vi "DataCSVFileRichInfo.vi"(9 "Language":u32, 11 "file path (dialog if empty)":path caption="文件路径 （空时为对话框）") -> (0 "路径输出":path, 1 "FileInfo":string, 2 "文件类型":string)   [LabVIEW 2015]
uses:
  <vilib>/regexp/Match Regular Expression.xnode
panel:
  out "判断":string
  out "末行":string
  out "数据首行":string
  out "行首":string
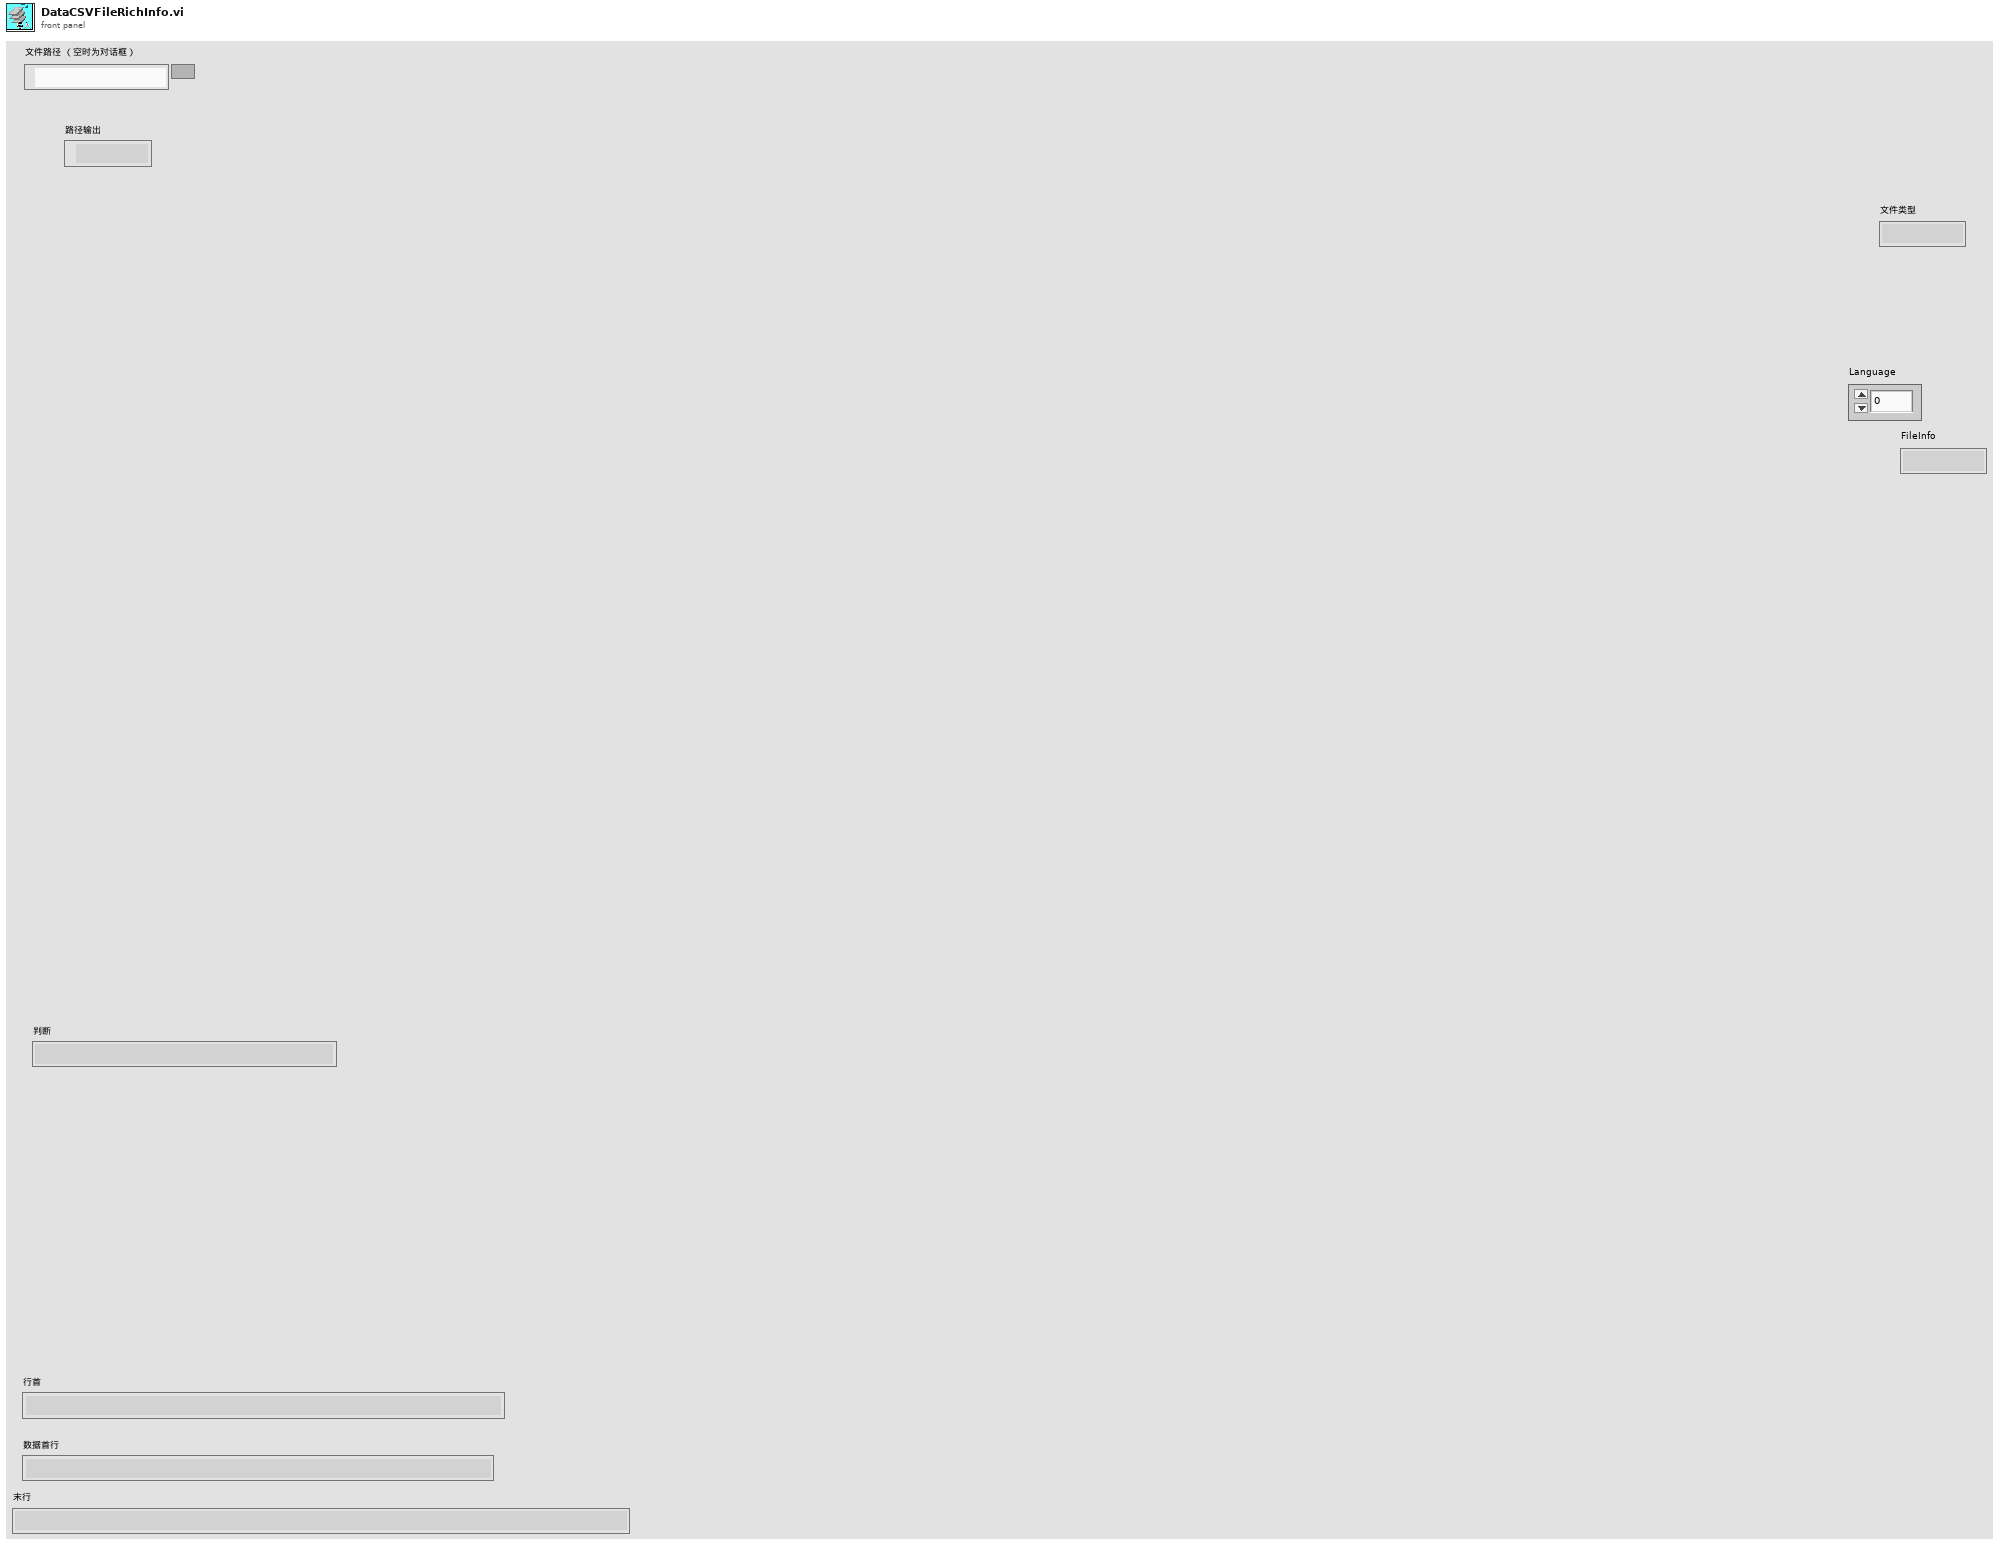
[diagram p1: front panel]
types:
  T1 = cluster{"基时间字符串":string, "基时间秒":dbl, "基时间标识":timestamp}
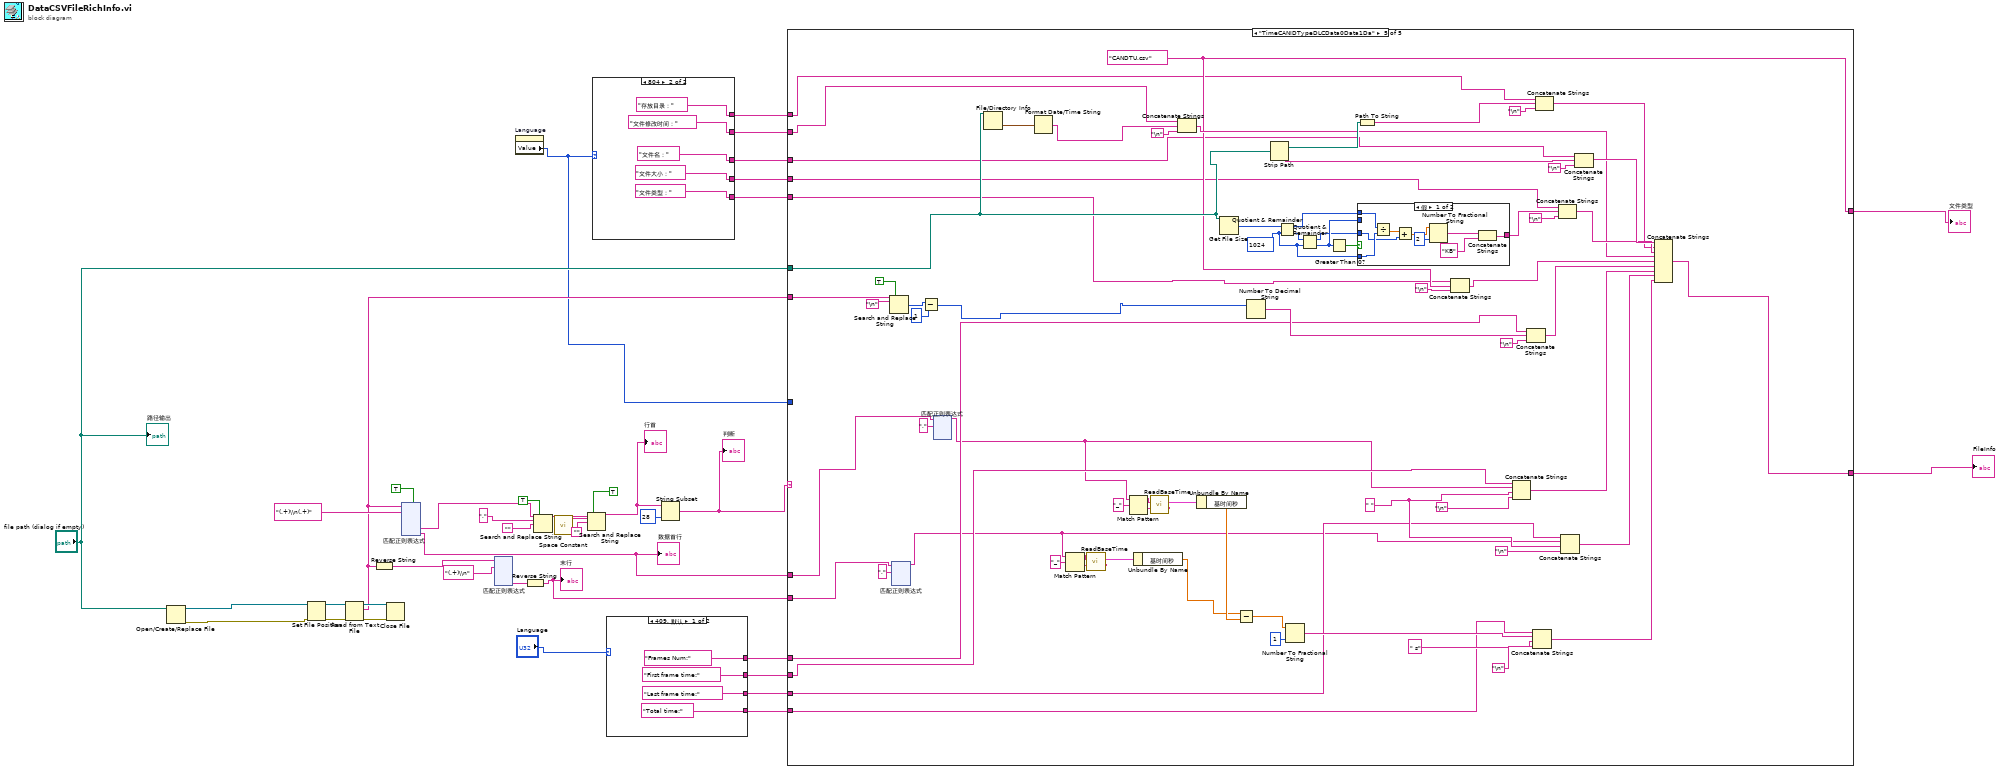
[diagram p0: block diagram]
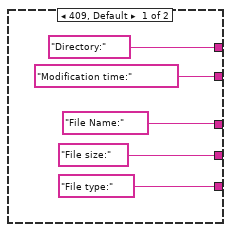
[diagram p2: hidden frame]
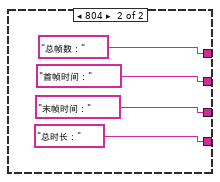
[diagram p3: hidden frame]
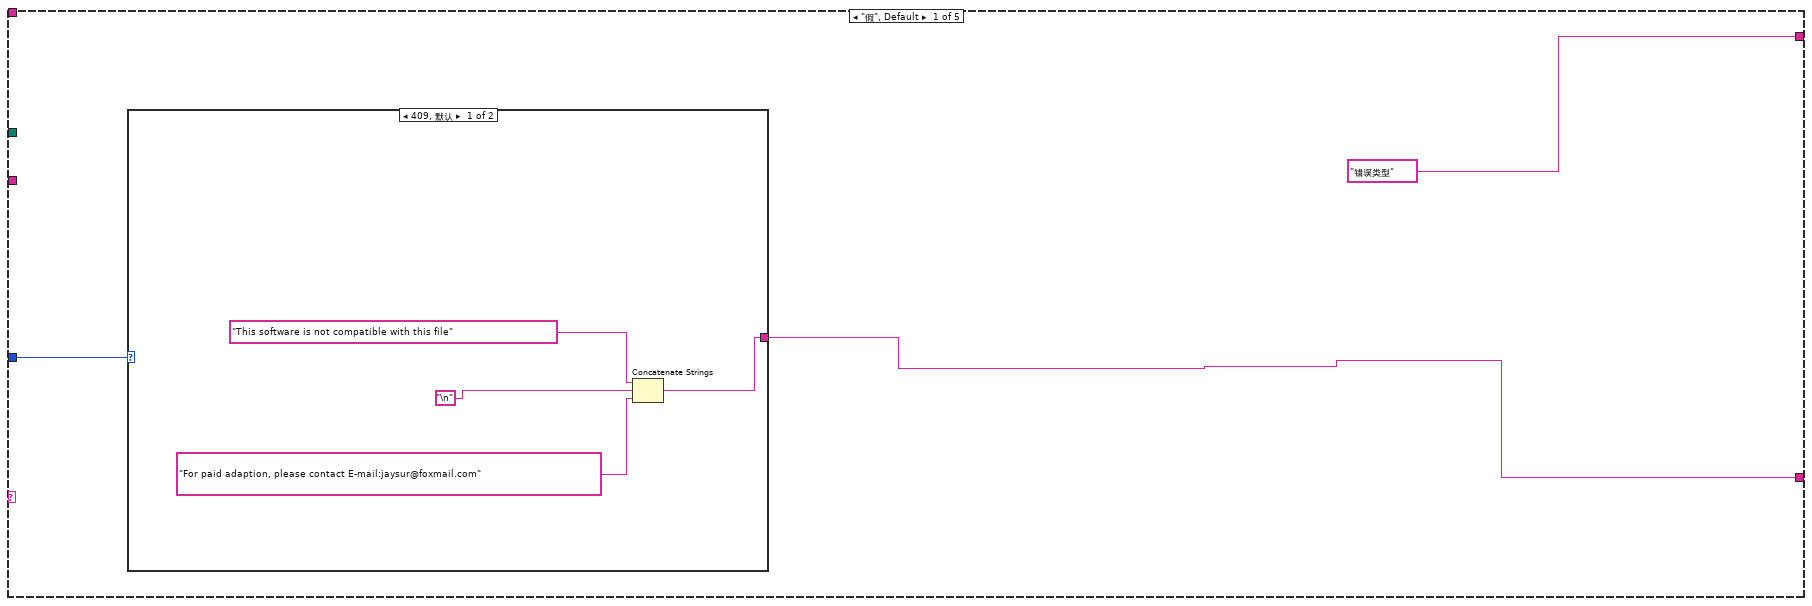
[diagram p4: hidden frame]
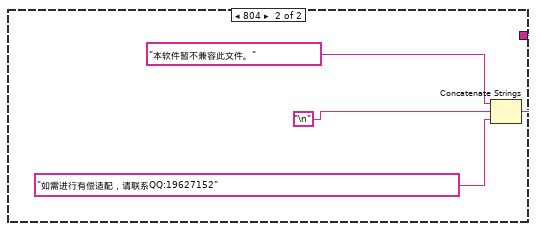
[diagram p5: hidden frame]
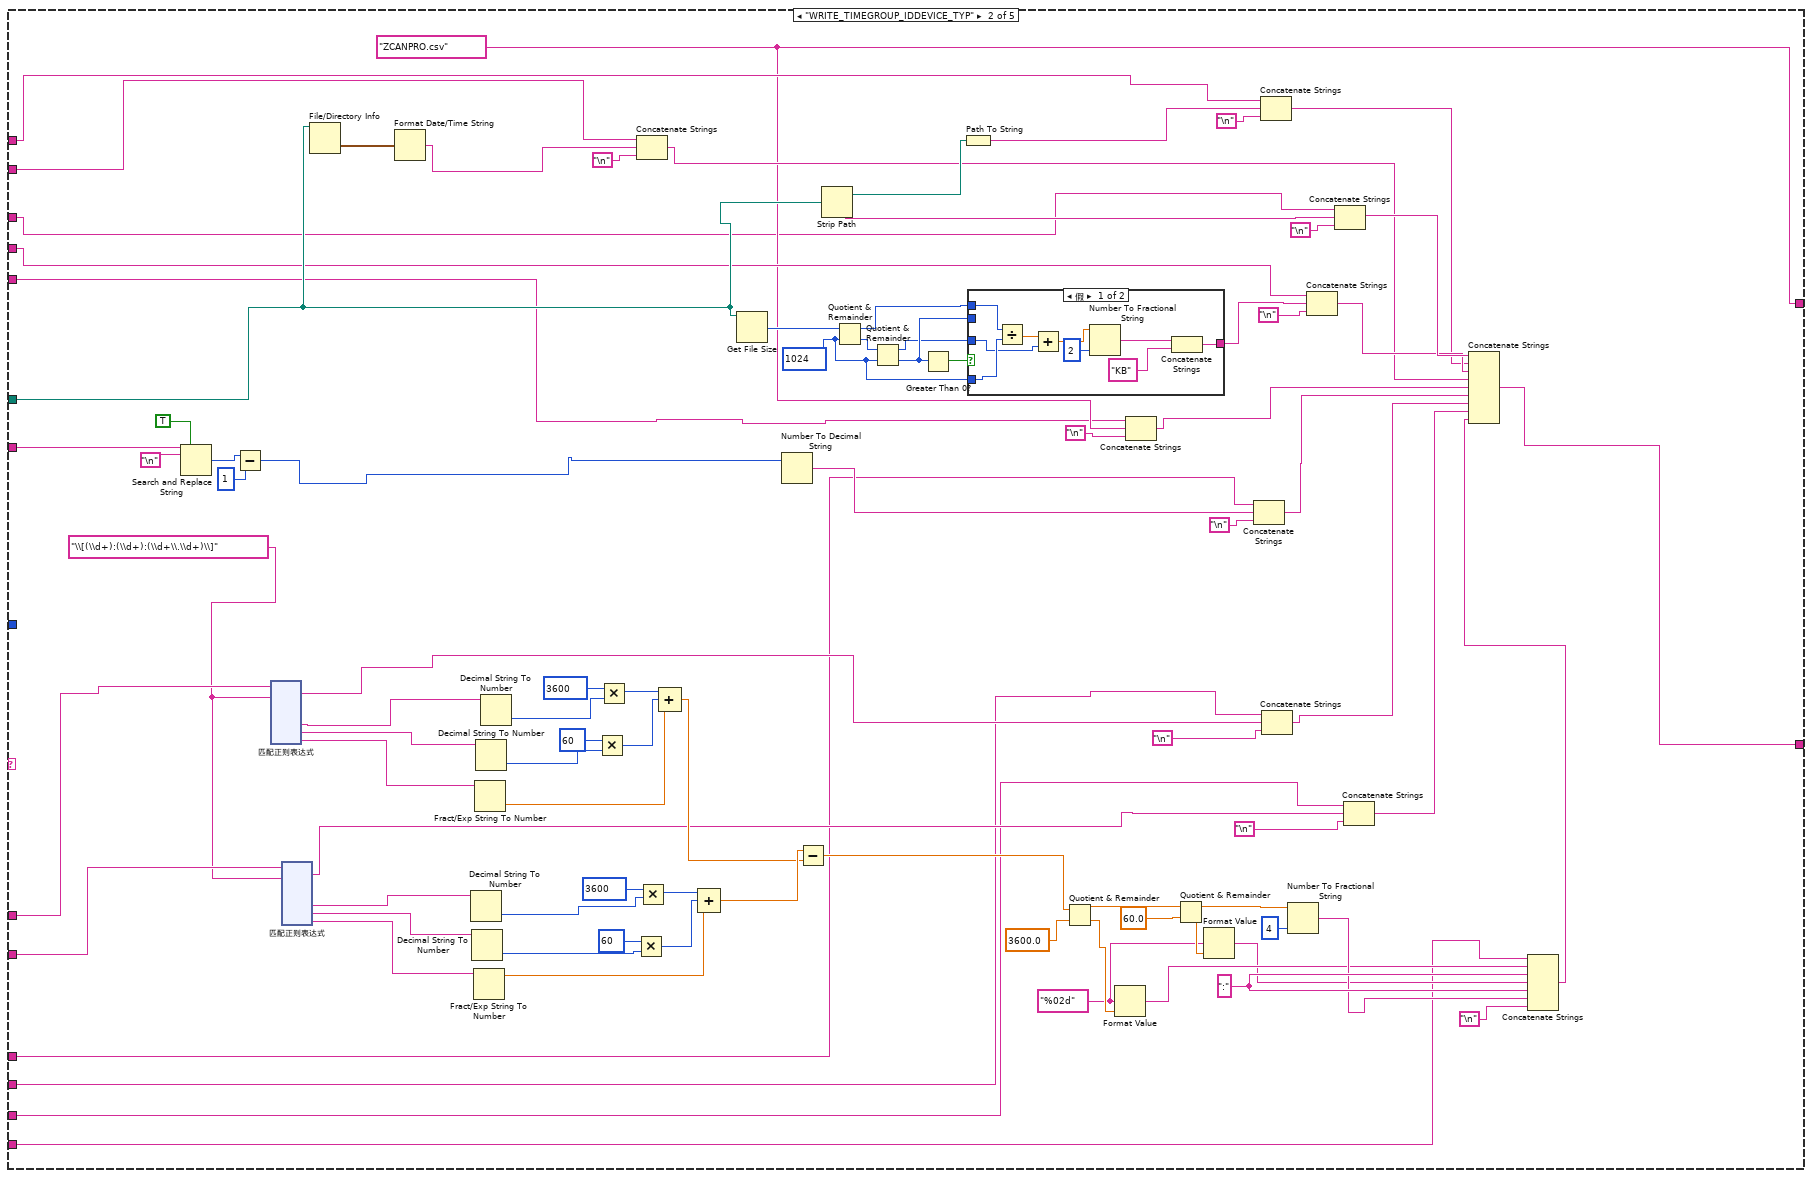
[diagram p6: hidden frame]
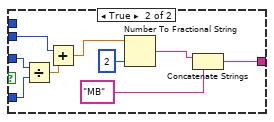
[diagram p7: hidden frame]
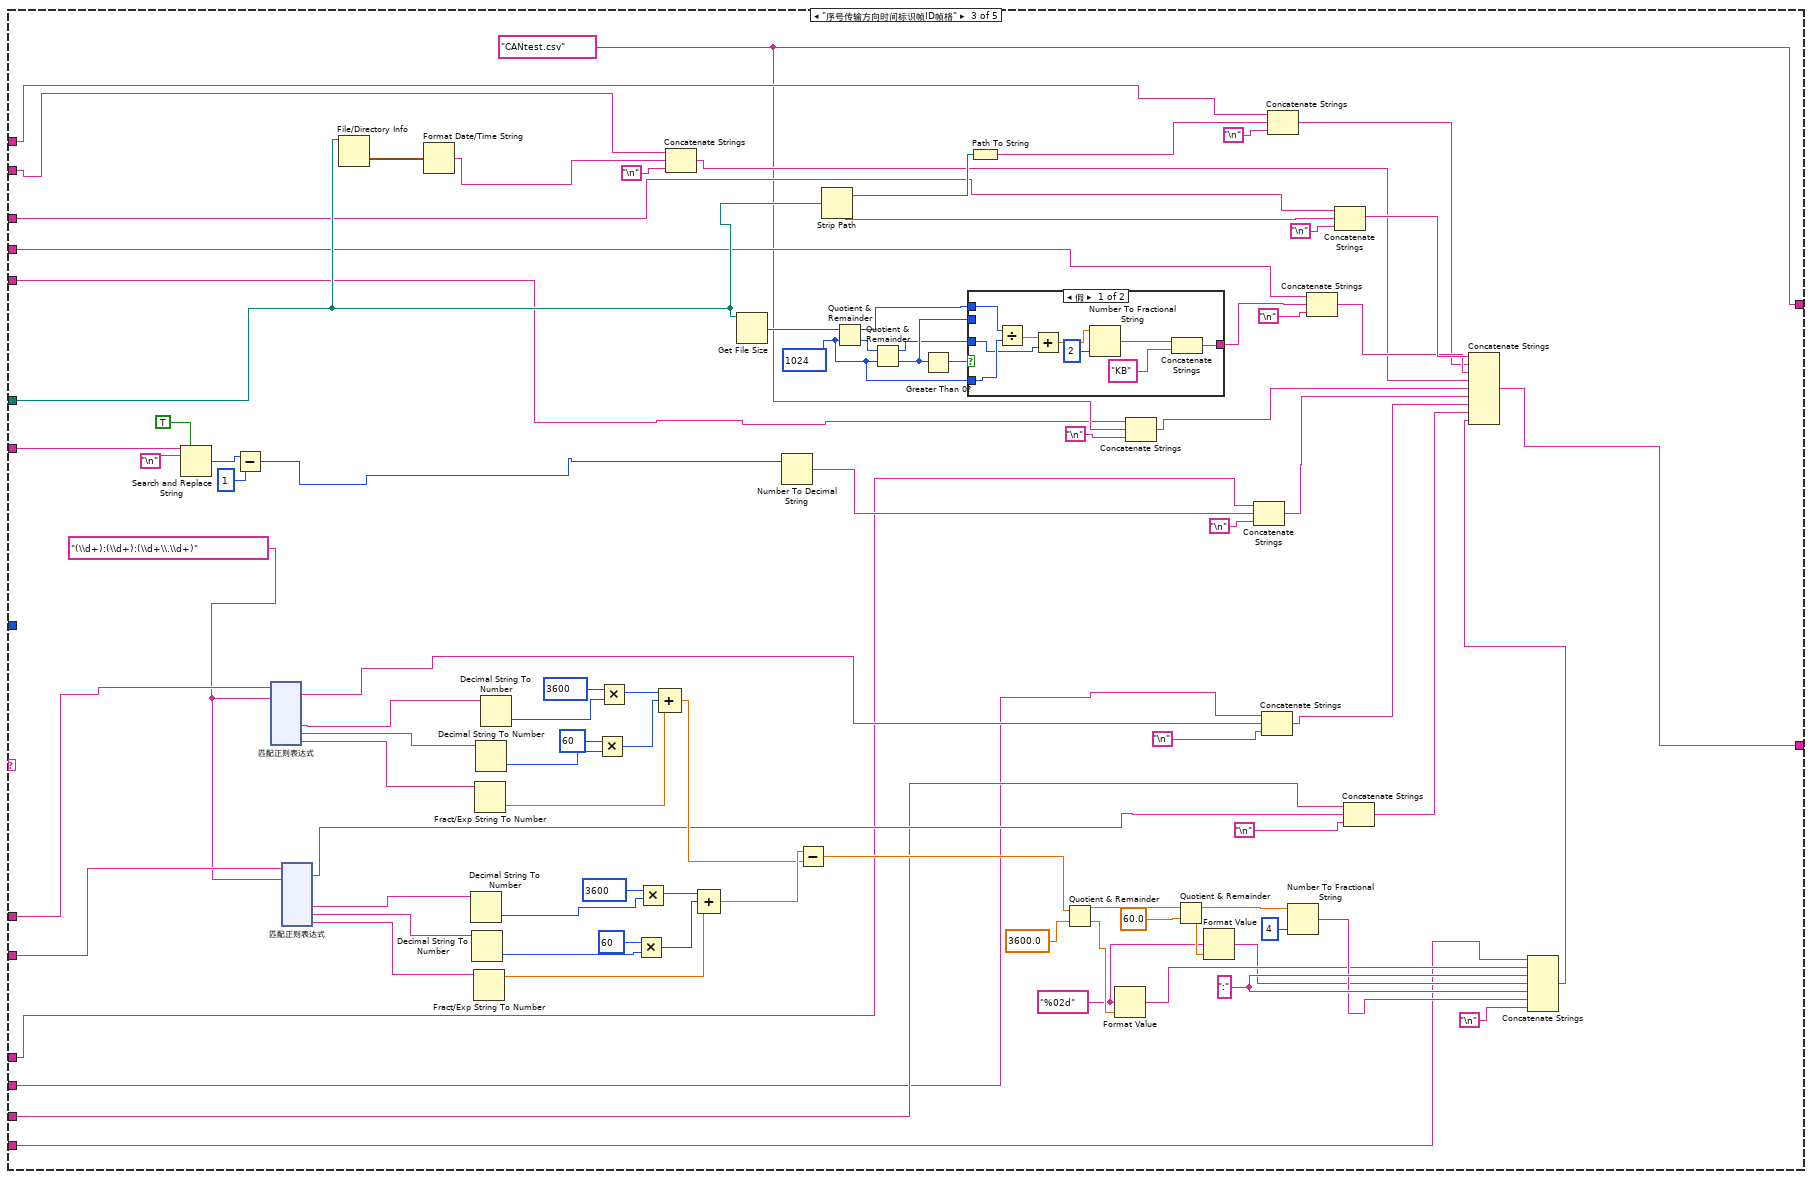
[diagram p8: hidden frame]
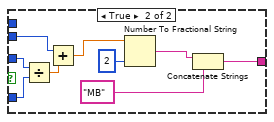
[diagram p9: hidden frame]
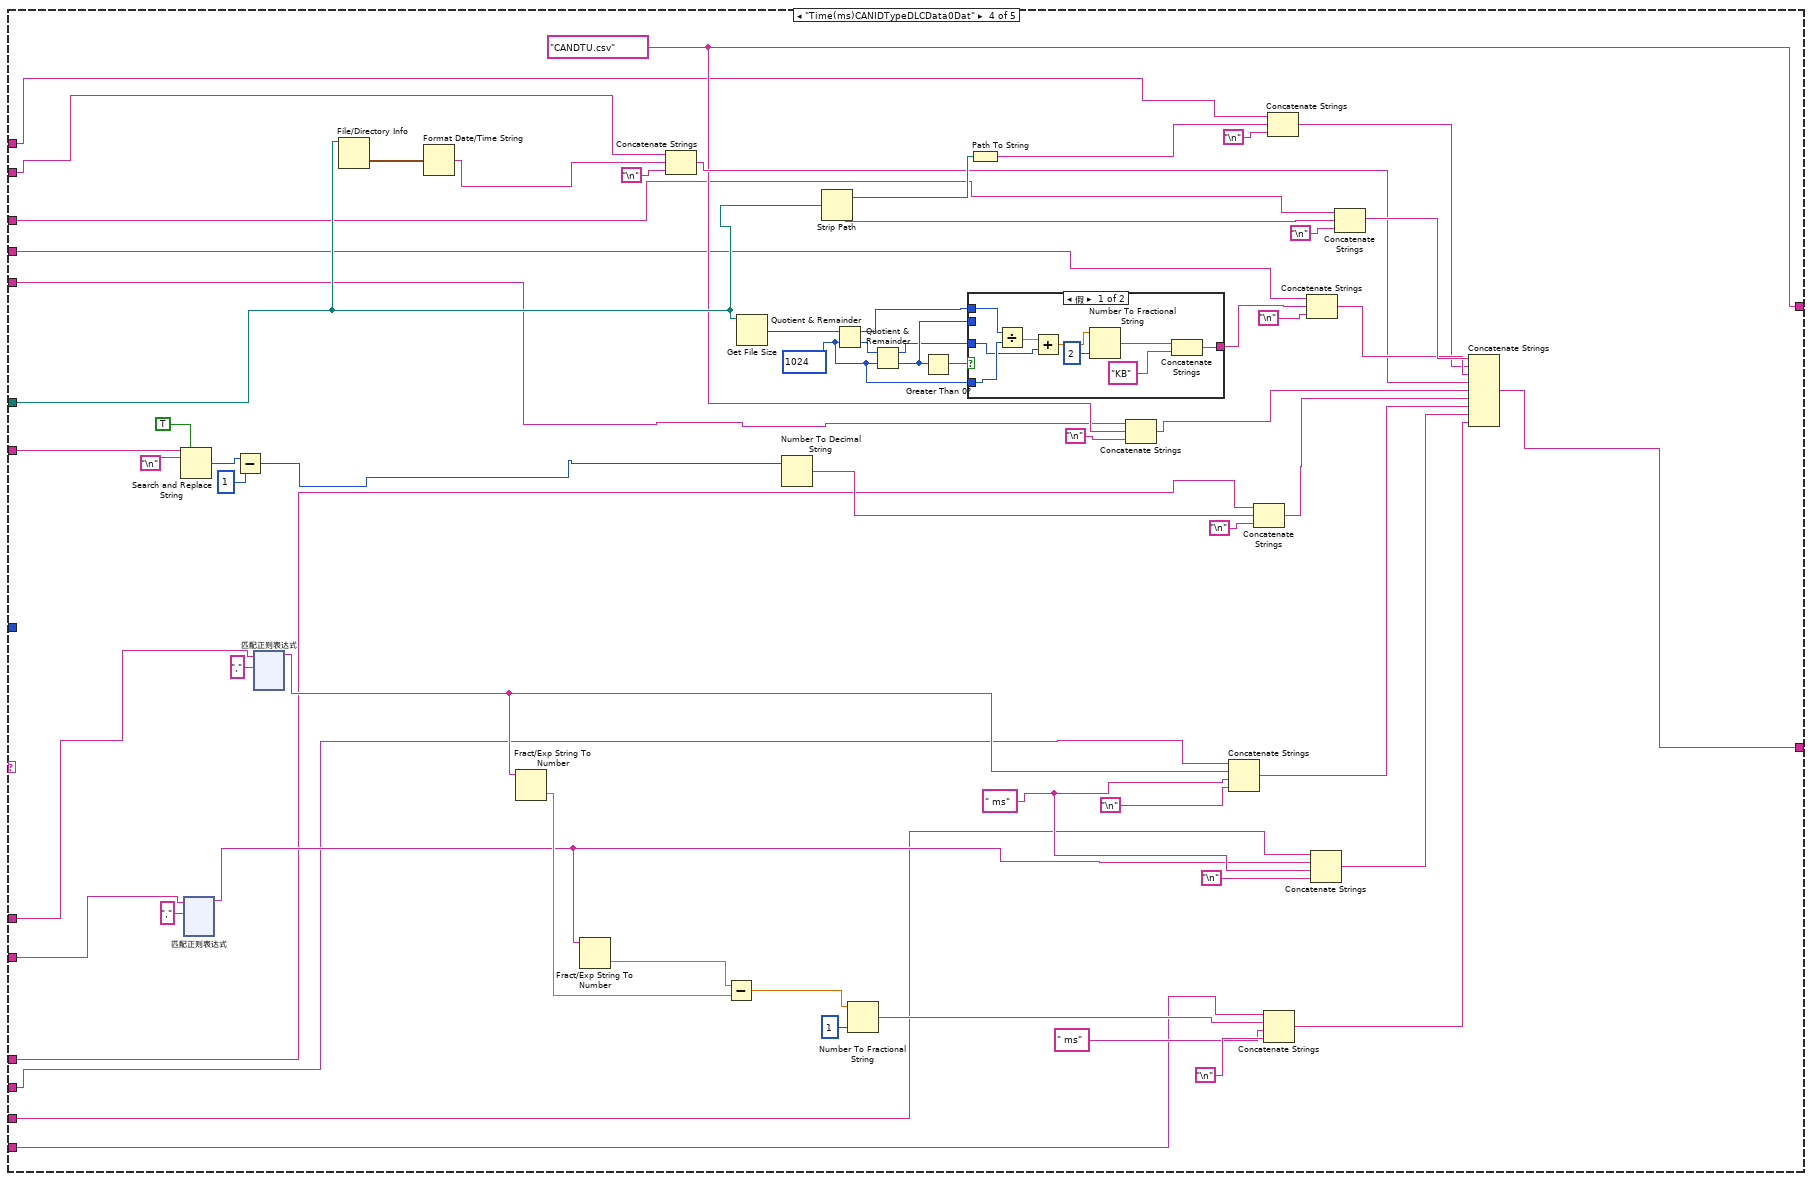
[diagram p10: hidden frame]
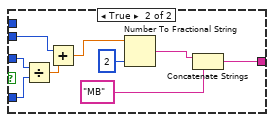
[diagram p11: hidden frame]
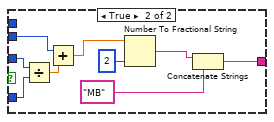
[diagram p12: hidden frame]
diagram:
  n1 = Open/Create/Replace File(file path (use dialog)="file path (dialog if empty)") -> (refnum out=w13:refnum<file>, error out=w12:errorcluster)  [unwired: 5 in, 1 out]
  n2 = Set File Position(refnum=w13, error in=w12) -> (refnum out=w37:refnum<file>, error out=w36:errorcluster)  [unwired: 2 in]
  n3 = Read from Text File(file (use dialog)=w37, error in=w36) -> (refnum out=w21:refnum<file>, text=w14:string, error out=w20:errorcluster)  [unwired: 2 in, 1 out]
  n4 = Reverse String(1:w14) -> (0:w25:string)
  n5 = Close File(refnum=w21, error in=w20) -> ()  [unwired: 2 out]
  n6 = xnode "匹配正则表达式"("输入字符串"=w14, "正则表达式"="(.+)\\n(.+)", "多行？(F)"=TRUE) -> ("子匹配 1"=w32:string, "子匹配 2"=w16:string)  [unwired: 3 in, 5 out]
  "数据首行" <- w16
  n7 = xnode "匹配正则表达式"("输入字符串"=w25, "正则表达式"="(.+)\\n") -> ("子匹配 1"=w24:string)  [unwired: 4 in, 5 out]
  n8 = property on="Language" class="DigNum (严格)"() -> ("Value"=w10:u32)  [unwired: 2 in, 2 out]
  n9 = Reverse String(1:w24) -> (0:w17:string)
  "末行" <- w17
  n10 = Search and Replace String(replace all?=TRUE ("替换全部？(F)"), input string=w32, search string=",", replace string="") -> (result string=w30:string)  [unwired: 4 in, 3 out]
  n11 = call <vilib>:"Space Constant.vi"() -> ("String"=w29:string)
  n12 = Search and Replace String(replace all?=TRUE ("替换全部？(F)"), input string=w30, search string=w29, replace string="") -> (result string=w23:string)  [unwired: 4 in, 3 out]
  "行首" <- w23
  n13 = case shown="804" w10 {
    tunnel: ["Modification time:" "文件修改时间："] -> w8
    tunnel: ["Directory:" "存放目录："] -> w9
    tunnel: ["File Name:" "文件名："] -> w7
    tunnel: ["File size:" "文件大小："] -> w6
    tunnel: ["File type:" "文件类型："] -> w5
    frame 409, Default {
    }
    frame 804 {
    }
  }
  n14 = case shown="409, 默认" "Language" {
    tunnel: ["Total time:" "总时长："] -> w4
    tunnel: ["Last frame time:" "末帧时间："] -> w3
    tunnel: ["First frame time:" "首帧时间："] -> w2
    tunnel: ["Frames Num:" "总帧数："] -> w1
    frame 409, Default {
    }
    frame 804 {
    }
  }
  n15 = String Subset(string=w23, length (rest)=28 ("长度（剩余）")) -> (substring=w15:string)  [unwired: 1 in]
  "判断" <- w15
  n16 = case shown="\"TimeCANIDTypeDLCData0Data1Da\"" w15 {
    tunnel: ["错误类型" w75 w418 w766 w1087] -> w39
    tunnel: [w59 w125 w469 w801 w1118] -> w38
    tunnel: "file path (dialog if empty)" -> [_ w80 w424 w787 w1104]
    tunnel: w17 -> [_ w93 w437 w772 w1091]
    tunnel: w16 -> [_ w92 w436 w773 w1092]
    tunnel: w14 -> [_ w117 w461 w796 w1113]
    tunnel: w10 -> [w58 _ _ _ _]
    tunnel: w9 -> [_ w77 w421 w762 w1083]
    tunnel: w8 -> [_ w78 w422 w761 w1082]
    tunnel: w7 -> [_ w73 w420 w763 w1084]
    tunnel: w6 -> [_ w76 w419 w764 w1085]
    tunnel: w5 -> [_ w74 w417 w765 w1086]
    tunnel: w4 -> [_ w72 w416 w757 w1078]
    tunnel: w3 -> [_ w71 w415 w758 w1079]
    tunnel: w2 -> [_ w70 w414 w760 w1081]
    tunnel: w1 -> [_ w69 w413 w759 w1080]
    frame "假", Default {
      n17 = case shown="409, 默认" w58 {
        tunnel: [w61 w65] -> w59
        frame 409, Default {
          n18 = Concatenate Strings("This software is not compatible with this file", "\n", "For paid adaption, please contact E-mail:jaysur@foxmail.com") -> (w61:string)
        }
        frame 804 {
          n19 = Concatenate Strings("本软件暂不兼容此文件。", "\n", "如需进行有偿适配，请联系QQ:19627152") -> (w65:string)
        }
      }
    }
    frame "WRITE_TIMEGROUP_IDDEVICE_TYP" {
      w88 = "\\[(\\d+):(\\d+):(\\d+\\.\\d+)\\]"
      w130 = i64 1024 ("y")
      w147 = "%02d" ("格式字符串")
      w153 = ":"
      w75 = "ZCANPRO.csv"
      n20 = Search and Replace String(replace all?=TRUE ("替换全部？(F)"), input string=w117, search string="\n") -> (number of replacements=w119:i32)  [unwired: 5 in, 3 out]
      n21 = Subtract(x=w119, y=1) -> (x-y=w116:i32)
      n22 = xnode "匹配正则表达式"("输入字符串"=w92, "正则表达式"=w88) -> ("所有匹配"=w89:string, "子匹配 1"=w115:string, "子匹配 2"=w114:string, "子匹配 3"=w113:string)  [unwired: 4 in, 4 out]
      n23 = xnode "匹配正则表达式"("输入字符串"=w93, "正则表达式"=w88) -> ("所有匹配"=w91:string, "子匹配 1"=w112:string, "子匹配 2"=w111:string, "子匹配 3"=w110:string)  [unwired: 4 in, 4 out]
      n24 = File/Directory Info(path=w80) -> (last mod=w83:timestamp)  [unwired: 1 in, 6 out]
      n25 = Format Date/Time String(seconds (now)=w83) -> (date/time string=w81:string)  [unwired: 2 in]
      n26 = Decimal String To Number(string=w112) -> (number=w98:i32)  [unwired: 2 in, 1 out]
      n27 = Decimal String To Number(string=w111) -> (number=w97:i32)  [unwired: 2 in, 1 out]
      n28 = Fract/Exp String To Number(string=w110) -> (number=w96:dbl)  [unwired: 3 in, 1 out]
      n29 = Fract/Exp String To Number(string=w113) -> (number=w103:dbl)  [unwired: 3 in, 1 out]
      n30 = Decimal String To Number(string=w114) -> (number=w109:i32)  [unwired: 2 in, 1 out]
      n31 = Decimal String To Number(string=w115) -> (number=w107:i32)  [unwired: 2 in, 1 out]
      n32 = Multiply(x=60, y=w109) -> (x*y=w104:i32)
      n33 = Multiply(x=3600, y=w107) -> (x*y=w105:i32)
      n34 = Multiply(x=60, y=w97) -> (x*y=w99:i32)
      n35 = Concatenate Strings(w78, w81, "\n") -> (w79:string)
      n36 = Multiply(x=3600, y=w98) -> (x*y=w100:i32)
      n37 = Compound Arithmetic op=ADD(w105, w104, w103) -> (w94:dbl)
      n38 = Compound Arithmetic op=ADD(w100, w99, w96) -> (w95:dbl)
      n39 = Get File Size(file=w80) -> (size (in bytes)=w133:i64)  [unwired: 1 in, 2 out]
      n40 = Number To Decimal String(number=w116) -> (decimal integer string=w136:string)  [unwired: 1 in]
      n41 = Subtract(x=w95, y=w94) -> (x-y=w90:dbl)
      n42 = Strip Path(path=w80) -> (stripped path=w85:path, name=w143:string)
      n43 = Quotient & Remainder(x=w133, y=w130) -> (x-y*floor(x/y)=w126:i64, floor(x/y)=w132:i64)
      n44 = Quotient & Remainder(x=w132, y=w130) -> (x-y*floor(x/y)=w128:i64, floor(x/y)=w129:i64)
      n45 = Greater Than 0?(x=w129) -> (x > 0?=w131:bool)
      n46 = Path To String(path=w85) -> (string=w86:string)
      n47 = case shown="假" w131 {
        tunnel: w130 -> [w400 w410]
        tunnel: w129 -> [_ w408]
        tunnel: w128 -> [w398 w411]
        tunnel: [w403 w406] -> w127
        tunnel: w126 -> [w401 _]
        frame False {
          n48 = Divide(x=w401, y=w400) -> (x/y=w399:dbl)
          n49 = Add(x=w399, y=w398) -> (x+y=w397:dbl)
          n50 = Number To Fractional String(number=w397, precision (6)=i16 2 ("精度(6)")) -> (F-format string=w395:string)  [unwired: 2 in]
          n51 = Concatenate Strings(w395, "KB" ("字符串")) -> (w403:string)
        }
        frame True {
          n52 = Divide(x=w411, y=w410) -> (x/y=w409:dbl)
          n53 = Add(x=w408, y=w409) -> (x+y=w407:dbl)
          n54 = Number To Fractional String(number=w407, precision (6)=i16 2 ("精度(6)")) -> (F-format string=w405:string)  [unwired: 2 in]
          n55 = Concatenate Strings(w405, "MB") -> (w406:string)
        }
      }
      n56 = Quotient & Remainder(x=w90, y=3600.0) -> (x-y*floor(x/y)=w157:dbl, floor(x/y)=w150:dbl)
      n57 = Format Value(format string=w147, value (0)=w150) -> (output string=w151:string)  [unwired: 1 in]
      n58 = Concatenate Strings(w74, w75, "\n") -> (w140:string)
      n59 = Quotient & Remainder(x=w157, y=60.0) -> (x-y*floor(x/y)=w155:dbl, floor(x/y)=w149:dbl)
      n60 = Format Value(format string=w147, value (0)=w149) -> (output string=w148:string)  [unwired: 1 in]
      n61 = Concatenate Strings(w69, w136, "\n") -> (w137:string)
      n62 = Concatenate Strings(w77, w86, "\n") -> (w84:string)
      n63 = Concatenate Strings(w70, w89, "\n") -> (w122:string)
      n64 = Number To Fractional String(number=w155, precision (6)=i16 4 ("精度(6)")) -> (F-format string=w152:string)  [unwired: 2 in]
      n65 = Concatenate Strings(w76, w127, "\n") -> (w134:string)
      n66 = Concatenate Strings(w73, w143, "\n") -> (w142:string)
      n67 = Concatenate Strings(w71, w91, "\n") -> (w123:string)
      n68 = Concatenate Strings(w72, w151, w153, w148, w153, w152, "\n") -> (w124:string)
      n69 = Concatenate Strings(w142, w84, w134, w79, w140, w137, w122, w123, w124) -> (w125:string)
    }
    frame "序号传输方向时间标识帧ID帧格" {
      w432 = "(\\d+):(\\d+):(\\d+\\.\\d+)"
      w474 = i64 1024 ("y")
      w491 = "%02d" ("格式字符串")
      w497 = ":"
      w418 = "CANtest.csv"
      n70 = Search and Replace String(replace all?=TRUE ("替换全部？(F)"), input string=w461, search string="\n") -> (number of replacements=w463:i32)  [unwired: 5 in, 3 out]
      n71 = Subtract(x=w463, y=1) -> (x-y=w460:i32)
      n72 = xnode "匹配正则表达式"("输入字符串"=w436, "正则表达式"=w432) -> ("所有匹配"=w433:string, "子匹配 1"=w459:string, "子匹配 2"=w458:string, "子匹配 3"=w457:string)  [unwired: 4 in, 4 out]
      n73 = xnode "匹配正则表达式"("输入字符串"=w437, "正则表达式"=w432) -> ("所有匹配"=w435:string, "子匹配 1"=w456:string, "子匹配 2"=w455:string, "子匹配 3"=w454:string)  [unwired: 4 in, 4 out]
      n74 = File/Directory Info(path=w424) -> (last mod=w427:timestamp)  [unwired: 1 in, 6 out]
      n75 = Format Date/Time String(seconds (now)=w427) -> (date/time string=w425:string)  [unwired: 2 in]
      n76 = Decimal String To Number(string=w456) -> (number=w442:i32)  [unwired: 2 in, 1 out]
      n77 = Decimal String To Number(string=w455) -> (number=w441:i32)  [unwired: 2 in, 1 out]
      n78 = Fract/Exp String To Number(string=w454) -> (number=w440:dbl)  [unwired: 3 in, 1 out]
      n79 = Fract/Exp String To Number(string=w457) -> (number=w447:dbl)  [unwired: 3 in, 1 out]
      n80 = Decimal String To Number(string=w458) -> (number=w453:i32)  [unwired: 2 in, 1 out]
      n81 = Decimal String To Number(string=w459) -> (number=w451:i32)  [unwired: 2 in, 1 out]
      n82 = Multiply(x=60, y=w453) -> (x*y=w448:i32)
      n83 = Multiply(x=3600, y=w451) -> (x*y=w449:i32)
      n84 = Multiply(x=60, y=w441) -> (x*y=w443:i32)
      n85 = Multiply(x=3600, y=w442) -> (x*y=w444:i32)
      n86 = Compound Arithmetic op=ADD(w449, w448, w447) -> (w438:dbl)
      n87 = Concatenate Strings(w422, w425, "\n") -> (w423:string)
      n88 = Compound Arithmetic op=ADD(w444, w443, w440) -> (w439:dbl)
      n89 = Get File Size(file=w424) -> (size (in bytes)=w477:i64)  [unwired: 1 in, 2 out]
      n90 = Number To Decimal String(number=w460) -> (decimal integer string=w480:string)  [unwired: 1 in]
      n91 = Subtract(x=w439, y=w438) -> (x-y=w434:dbl)
      n92 = Strip Path(path=w424) -> (stripped path=w429:path, name=w487:string)
      n93 = Quotient & Remainder(x=w477, y=w474) -> (x-y*floor(x/y)=w470:i64, floor(x/y)=w476:i64)
      n94 = Quotient & Remainder(x=w476, y=w474) -> (x-y*floor(x/y)=w472:i64, floor(x/y)=w473:i64)
      n95 = Greater Than 0?(x=w473) -> (x > 0?=w475:bool)
      n96 = case shown="假" w475 {
        tunnel: w474 -> [w744 w754]
        tunnel: w473 -> [_ w752]
        tunnel: w472 -> [w742 w755]
        tunnel: [w747 w750] -> w471
        tunnel: w470 -> [w745 _]
        frame False {
          n97 = Divide(x=w745, y=w744) -> (x/y=w743:dbl)
          n98 = Add(x=w743, y=w742) -> (x+y=w741:dbl)
          n99 = Number To Fractional String(number=w741, precision (6)=i16 2 ("精度(6)")) -> (F-format string=w739:string)  [unwired: 2 in]
          n100 = Concatenate Strings(w739, "KB" ("字符串")) -> (w747:string)
        }
        frame True {
          n101 = Divide(x=w755, y=w754) -> (x/y=w753:dbl)
          n102 = Add(x=w752, y=w753) -> (x+y=w751:dbl)
          n103 = Number To Fractional String(number=w751, precision (6)=i16 2 ("精度(6)")) -> (F-format string=w749:string)  [unwired: 2 in]
          n104 = Concatenate Strings(w749, "MB") -> (w750:string)
        }
      }
      n105 = Path To String(path=w429) -> (string=w430:string)
      n106 = Quotient & Remainder(x=w434, y=3600.0) -> (x-y*floor(x/y)=w501:dbl, floor(x/y)=w494:dbl)
      n107 = Format Value(format string=w491, value (0)=w494) -> (output string=w495:string)  [unwired: 1 in]
      n108 = Concatenate Strings(w417, w418, "\n") -> (w484:string)
      n109 = Quotient & Remainder(x=w501, y=60.0) -> (x-y*floor(x/y)=w499:dbl, floor(x/y)=w493:dbl)
      n110 = Format Value(format string=w491, value (0)=w493) -> (output string=w492:string)  [unwired: 1 in]
      n111 = Concatenate Strings(w413, w480, "\n") -> (w481:string)
      n112 = Concatenate Strings(w414, w433, "\n") -> (w466:string)
      n113 = Concatenate Strings(w421, w430, "\n") -> (w428:string)
      n114 = Number To Fractional String(number=w499, precision (6)=i16 4 ("精度(6)")) -> (F-format string=w496:string)  [unwired: 2 in]
      n115 = Concatenate Strings(w419, w471, "\n") -> (w478:string)
      n116 = Concatenate Strings(w420, w487, "\n") -> (w486:string)
      n117 = Concatenate Strings(w415, w435, "\n") -> (w467:string)
      n118 = Concatenate Strings(w416, w495, w497, w492, w497, w496, "\n") -> (w468:string)
      n119 = Concatenate Strings(w486, w428, w478, w423, w484, w481, w466, w467, w468) -> (w469:string)
    }
    frame "Time(ms)CANIDTypeDLCData0Dat" {
      w780 = " ms"
      w806 = i64 1024 ("y")
      w766 = "CANDTU.csv"
      n120 = Search and Replace String(replace all?=TRUE ("替换全部？(F)"), input string=w796, search string="\n") -> (number of replacements=w798:i32)  [unwired: 5 in, 3 out]
      n121 = xnode "匹配正则表达式"("输入字符串"=w772, "正则表达式"=",") -> ("匹配之前"=w768:string)  [unwired: 4 in, 4 out]
      n122 = Subtract(x=w798, y=1) -> (x-y=w795:i32)
      n123 = xnode "匹配正则表达式"("输入字符串"=w773, "正则表达式"=",") -> ("匹配之前"=w767:string)  [unwired: 4 in, 4 out]
      n124 = File/Directory Info(path=w787) -> (last mod=w790:timestamp)  [unwired: 1 in, 6 out]
      n125 = Format Date/Time String(seconds (now)=w790) -> (date/time string=w788:string)  [unwired: 2 in]
      n126 = Fract/Exp String To Number(string=w767) -> (number=w778:dbl)  [unwired: 3 in, 1 out]
      n127 = Fract/Exp String To Number(string=w768) -> (number=w779:dbl)  [unwired: 3 in, 1 out]
      n128 = Concatenate Strings(w761, w788, "\n") -> (w786:string)
      n129 = Subtract(x=w779, y=w778) -> (x-y=w777:dbl)
      n130 = Get File Size(file=w787) -> (size (in bytes)=w809:i64)  [unwired: 1 in, 2 out]
      n131 = Number To Decimal String(number=w795) -> (decimal integer string=w812:string)  [unwired: 1 in]
      n132 = Strip Path(path=w787) -> (stripped path=w792:path, name=w819:string)
      n133 = Quotient & Remainder(x=w809, y=w806) -> (x-y*floor(x/y)=w802:i64, floor(x/y)=w808:i64)
      n134 = Number To Fractional String(number=w777, precision (6)=i16 1 ("精度(6)")) -> (F-format string=w775:string)  [unwired: 2 in]
      n135 = Quotient & Remainder(x=w808, y=w806) -> (x-y*floor(x/y)=w804:i64, floor(x/y)=w805:i64)
      n136 = Greater Than 0?(x=w805) -> (x > 0?=w807:bool)
      n137 = case shown="假" w807 {
        tunnel: w806 -> [w1053 w1063]
        tunnel: w805 -> [_ w1061]
        tunnel: w804 -> [w1051 w1064]
        tunnel: [w1056 w1059] -> w803
        tunnel: w802 -> [w1054 _]
        frame False {
          n138 = Divide(x=w1054, y=w1053) -> (x/y=w1052:dbl)
          n139 = Add(x=w1052, y=w1051) -> (x+y=w1050:dbl)
          n140 = Number To Fractional String(number=w1050, precision (6)=i16 2 ("精度(6)")) -> (F-format string=w1048:string)  [unwired: 2 in]
          n141 = Concatenate Strings(w1048, "KB" ("字符串")) -> (w1056:string)
        }
        frame True {
          n142 = Divide(x=w1064, y=w1063) -> (x/y=w1062:dbl)
          n143 = Add(x=w1061, y=w1062) -> (x+y=w1060:dbl)
          n144 = Number To Fractional String(number=w1060, precision (6)=i16 2 ("精度(6)")) -> (F-format string=w1058:string)  [unwired: 2 in]
          n145 = Concatenate Strings(w1058, "MB") -> (w1059:string)
        }
      }
      n146 = Path To String(path=w792) -> (string=w793:string)
      n147 = Concatenate Strings(w765, w766, "\n") -> (w816:string)
      n148 = Concatenate Strings(w760, w767, w780, "\n") -> (w771:string)
      n149 = Concatenate Strings(w759, w812, "\n") -> (w813:string)
      n150 = Concatenate Strings(w757, w775, " ms", "\n") -> (w769:string)
      n151 = Concatenate Strings(w762, w793, "\n") -> (w791:string)
      n152 = Concatenate Strings(w764, w803, "\n") -> (w810:string)
      n153 = Concatenate Strings(w758, w768, w780, "\n") -> (w770:string)
      n154 = Concatenate Strings(w763, w819, "\n") -> (w818:string)
      n155 = Concatenate Strings(w818, w791, w810, w786, w816, w813, w771, w770, w769) -> (w801:string)
    }
    frame "TimeCANIDTypeDLCData0Data1Da" {
      w1097 = " "
      w1123 = i64 1024 ("y")
      w1087 = "CANDTU.csv"
      n156 = Search and Replace String(replace all?=TRUE ("替换全部？(F)"), input string=w1113, search string="\n") -> (number of replacements=w1115:i32)  [unwired: 5 in, 3 out]
      n157 = xnode "匹配正则表达式"("输入字符串"=w1091, "正则表达式"=",") -> ("匹配之前"=w1067:string)  [unwired: 4 in, 4 out]
      n158 = Subtract(x=w1115, y=1) -> (x-y=w1112:i32)
      n159 = xnode "匹配正则表达式"("输入字符串"=w1092, "正则表达式"=",") -> ("匹配之前"=w1073:string)  [unwired: 4 in, 4 out]
      n160 = File/Directory Info(path=w1104) -> (last mod=w1107:timestamp)  [unwired: 1 in, 6 out]
      n161 = Format Date/Time String(seconds (now)=w1107) -> (date/time string=w1105:string)  [unwired: 2 in]
      n162 = Match Pattern(string=w1067, regular expression="_" ("正则表达式")) -> (before substring=w1070:string, after substring=w1069:string)  [unwired: 1 in, 2 out]
      n163 = call "ReadBaseTime.vi"("时间字符"=w1069, "日期字符"=w1070) -> ("基时间簇"=w1068:T1)  [unwired: 7 in]
      n164 = Match Pattern(string=w1073, regular expression="_" ("正则表达式")) -> (before substring=w1076:string, after substring=w1075:string)  [unwired: 1 in, 2 out]
      n165 = Unbundle By Name(w1068) -> ("基时间秒"=w1066:dbl)
      n166 = call "ReadBaseTime.vi"("时间字符"=w1075, "日期字符"=w1076) -> ("基时间簇"=w1074:T1)  [unwired: 7 in]
      n167 = Concatenate Strings(w1082, w1105, "\n") -> (w1103:string)
      n168 = Unbundle By Name(w1074) -> ("基时间秒"=w1072:dbl)
      n169 = Get File Size(file=w1104) -> (size (in bytes)=w1126:i64)  [unwired: 1 in, 2 out]
      n170 = Subtract(x=w1066, y=w1072) -> (x-y=w1096:dbl)
      n171 = Number To Decimal String(number=w1112) -> (decimal integer string=w1129:string)  [unwired: 1 in]
      n172 = Strip Path(path=w1104) -> (stripped path=w1109:path, name=w1136:string)
      n173 = Quotient & Remainder(x=w1126, y=w1123) -> (x-y*floor(x/y)=w1119:i64, floor(x/y)=w1125:i64)
      n174 = Number To Fractional String(number=w1096, precision (6)=i16 1 ("精度(6)")) -> (F-format string=w1094:string)  [unwired: 2 in]
      n175 = Quotient & Remainder(x=w1125, y=w1123) -> (x-y*floor(x/y)=w1121:i64, floor(x/y)=w1122:i64)
      n176 = Greater Than 0?(x=w1122) -> (x > 0?=w1124:bool)
      n177 = case shown="假" w1124 {
        tunnel: w1123 -> [w1370 w1380]
        tunnel: w1122 -> [_ w1378]
        tunnel: w1121 -> [w1368 w1381]
        tunnel: [w1373 w1376] -> w1120
        tunnel: w1119 -> [w1371 _]
        frame False {
          n178 = Divide(x=w1371, y=w1370) -> (x/y=w1369:dbl)
          n179 = Add(x=w1369, y=w1368) -> (x+y=w1367:dbl)
          n180 = Number To Fractional String(number=w1367, precision (6)=i16 2 ("精度(6)")) -> (F-format string=w1365:string)  [unwired: 2 in]
          n181 = Concatenate Strings(w1365, "KB" ("字符串")) -> (w1373:string)
        }
        frame True {
          n182 = Divide(x=w1381, y=w1380) -> (x/y=w1379:dbl)
          n183 = Add(x=w1378, y=w1379) -> (x+y=w1377:dbl)
          n184 = Number To Fractional String(number=w1377, precision (6)=i16 2 ("精度(6)")) -> (F-format string=w1375:string)  [unwired: 2 in]
          n185 = Concatenate Strings(w1375, "MB") -> (w1376:string)
        }
      }
      n186 = Path To String(path=w1109) -> (string=w1110:string)
      n187 = Concatenate Strings(w1086, w1087, "\n") -> (w1133:string)
      n188 = Concatenate Strings(w1081, w1073, w1097, "\n") -> (w1090:string)
      n189 = Concatenate Strings(w1080, w1129, "\n") -> (w1130:string)
      n190 = Concatenate Strings(w1078, w1094, " s", "\n") -> (w1088:string)
      n191 = Concatenate Strings(w1083, w1110, "\n") -> (w1108:string)
      n192 = Concatenate Strings(w1085, w1120, "\n") -> (w1127:string)
      n193 = Concatenate Strings(w1079, w1067, w1097, "\n") -> (w1089:string)
      n194 = Concatenate Strings(w1084, w1136, "\n") -> (w1135:string)
      n195 = Concatenate Strings(w1135, w1108, w1127, w1103, w1133, w1130, w1090, w1089, w1088) -> (w1118:string)
    }
  }
  "FileInfo" <- w38
  "文件类型" <- w39
  "路径输出" <- "file path (dialog if empty)"
